vi "Destroy Return FIFO.vi"(8 "error in (no error)":errorcluster, 11 "Transfer Group in":refnum<class "Transfer Group.lvclass">) -> (0 "error out":errorcluster, 3 "Transfer Group out":refnum<class "Transfer Group.lvclass">)   [LabVIEW 2021, in "DSF Core.lvlib" / "Transfer Group.lvclass"]
uses:
  Transfer Group.lvclass
  Transfer Group.lvclass/Transfer Group.ctl
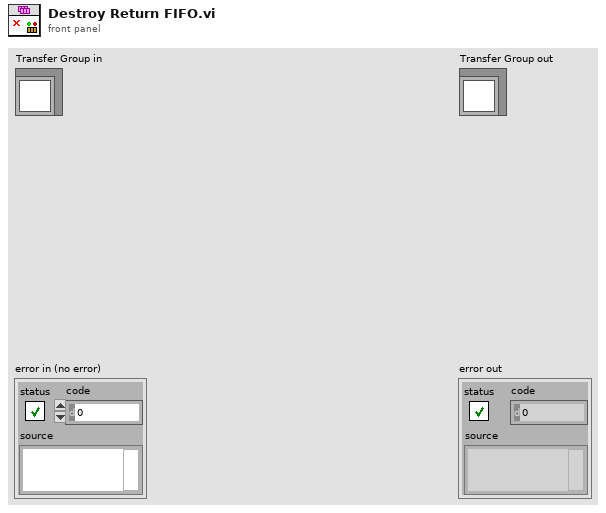
[diagram p1: front panel]
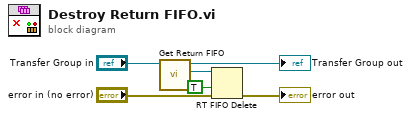
[diagram p0: block diagram]
diagram:
  n1 = call "Get Return FIFO.vi"("Transfer Group in"="Transfer Group in") -> ("Return FIFO"=w3:refnum<k33>, "Transfer Group out"=→"Transfer Group out":refnum<class "Transfer Group.lvclass">)  [unwired: 9 in]
  n2 = RT FIFO Delete(0:w3, 2:TRUE ("force destroy? (F)"), 3:"error in (no error)") -> (11:→"error out":errorcluster)
